vi "incrementPolarity.vi"(1 "inc(mm)":dbl, 2 "initPos":dbl, 3 "finPos":dbl) -> (0 "polInc (mm)":dbl=0.9020000000000001)   [LabVIEW 2015]
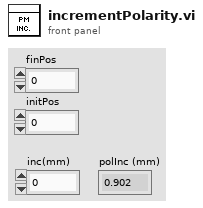
[diagram p1: front panel]
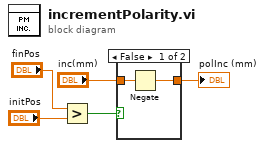
[diagram p0: block diagram]
diagram:
  n1 = Greater?(x="finPos", y="initPos") -> (0:w4:bool)
  n2 = case shown="False" w4 {
    tunnel: "inc(mm)" -> [w6 w8]
    tunnel: [w7 w8] -> w5
    frame False {
      n3 = Negate(x=w6) -> (-x=w7:dbl)
    }
    frame True {
    }
  }
  "polInc (mm)" <- w5
